vi "Gen_Func.vi"() -> ()   [LabVIEW 2021]
panel:
  in  "Amplitud":dbl(knob) scale=0.0..10.0
  in  "Offset":dbl(knob) scale=0.0..10.0
  in  "DC":dbl(knob) scale=0.0..10.0
  out "x+y":dbl
  in  "Enum":T1(ring)
  out "Waveform Chart":dbl(graph)
  in  "Stop":bool
  # "Mendoza Meza Manuel Everardo \n  GENERADOR DE FUNCIONES"
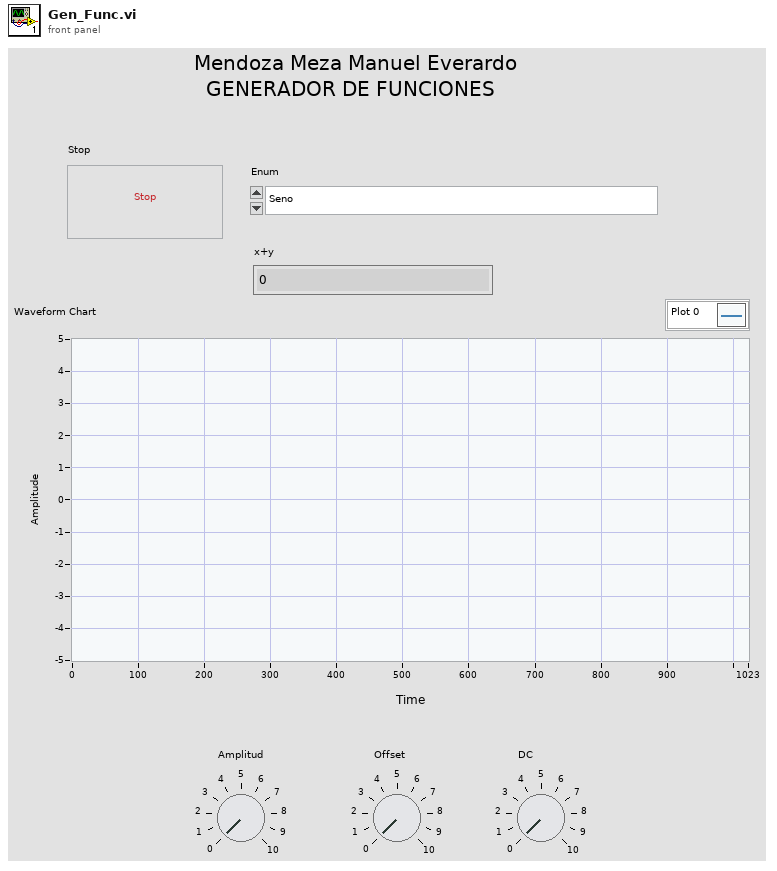
[diagram p1: front panel]
types:
  T1 = enum16{"Seno", "Pulso", "Triangular", "Diente de sierra", "Tangente", "GND", "DC"}
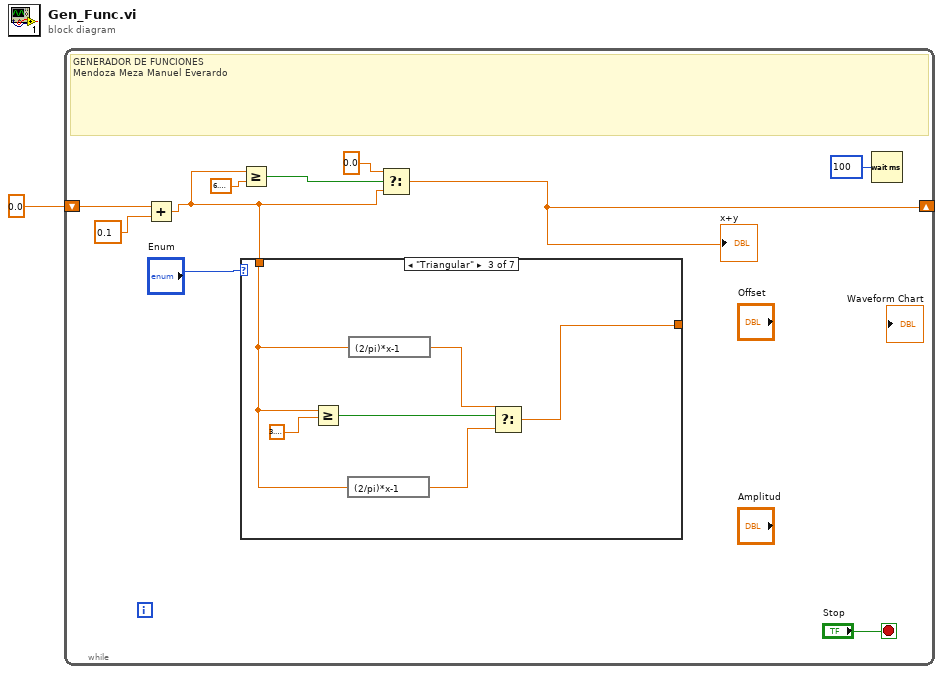
[diagram p0: block diagram]
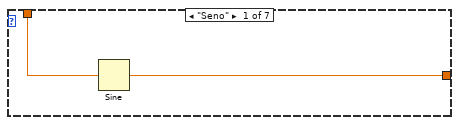
[diagram p2: hidden frame]
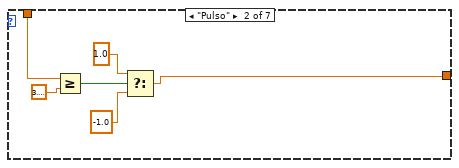
[diagram p3: hidden frame]
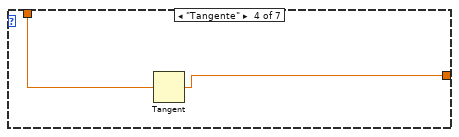
[diagram p4: hidden frame]
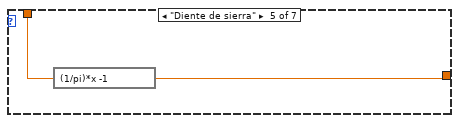
[diagram p5: hidden frame]
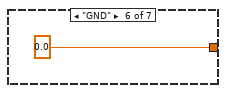
[diagram p6: hidden frame]
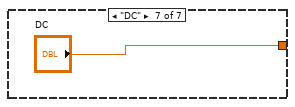
[diagram p7: hidden frame]
diagram:
  n1 = while {
    shift-right: [w3] -> _
    shift-left: 0.0 -> [w7]
    stop <- "Stop" stop-if-true
    # "GENERADOR DE FUNCIONES\nMendoza Meza Manuel Everardo"
    n2 = Add(x=w7, y=0.1) -> (x+y=w2:dbl)
    n3 = Greater Or Equal?(x=w2, y=6.283185307179586) -> (x >= y?=w5:bool)
    n4 = case shown="\"Triangular\"" "Enum" {
      tunnel: w2 -> [w13 w18 w22 w26 w29 _ _]
      tunnel: [w12 w14 w20 w27 w28 0.0 ("f") "DC"] -> _
      frame "Seno" {
        n5 = Sine(x=w13) -> (sin(x)=w12:dbl)
      }
      frame "Pulso" {
        n6 = Greater Or Equal?(x=w18, y=3.141592653589793) -> (x >= y?=w15:bool)
        n7 = Select(t=1.0, s=w15, f=-1.0) -> (s? t:f=w14:dbl)
      }
      frame "Triangular" {
        n8 = Greater Or Equal?(x=w22, y=3.141592653589793) -> (x >= y?=w21:bool)
        n9 = expression code="(2/pi)*x-1"(w22) -> (w23:dbl)
        n10 = expression code="(2/pi)*x-1"(w22) -> (w24:dbl)
        n11 = Select(t=w24, s=w21, f=w23) -> (s? t:f=w20:dbl)
      }
      frame "Tangente" {
        n12 = Tangent(1:w26) -> (0:w27:dbl)
      }
      frame "Diente de sierra" {
        n13 = expression code="(1/pi)*x -1"(w29) -> (w28:dbl)
      }
      frame "GND" {
      }
      frame "DC" {
      }
    }
    n14 = Select(t=0.0, s=w5, f=w2) -> (s? t:f=w3:dbl)
    "x+y" <- w3
    n15 = Wait (ms)(milliseconds to wait=u32 100) -> ()  [unwired: 1 out]
  }
